vi "CreatePopupWindow.vi"(5 "Offset_y":i32, 6 "Flags (SDL_WINDOW_TOOLTIP)":T1=262144 items=["0"=0, "SDL_WINDOW_FULLSCREEN"=1, "SDL_WINDOW_OPENGL"=2, "SDL_WINDOW_OCCLUDED"=4, "SDL_WINDOW_HIDDEN"=8, "SDL_WINDOW_BORDERLESS"=16, "SDL_WINDOW_RESIZABLE"=32, "SDL_WINDOW_MINIMIZED"=64, "SDL_WINDOW_MAXIMIZED"=128, "SDL_WINDOW_MOUSE_GRABBED"=256, "SDL_WINDOW_INPUT_FOCUS"=512, "SDL_WINDOW_MOUSE_FOCUS"=1024, "SDL_WINDOW_EXTERNAL"=2048, "SDL_WINDOW_MODAL"=4096, "SDL_WINDOW_HIGH_PIXEL_DENSITY"=8192, "SDL_WINDOW_MOUSE_CAPTURE"=16384, "SDL_WINDOW_MOUSE_RELATIVE_MODE"=32768, "SDL_WINDOW_ALWAYS_ON_TOP"=65536, "SDL_WINDOW_UTILITY"=131072, "SDL_WINDOW_TOOLTIP"=262144, "SDL_WINDOW_POPUP_MENU"=524288, "SDL_WINDOW_KEYBOARD_GRABBED"=1048576, "SDL_WINDOW_VULKAN"=268435456, "SDL_WINDOW_METAL"=536870912, "SDL_WINDOW_TRANSPARENT"=1073741824, "SDL_WINDOW_NOT_FOCUSABLE"=2147483648], 7 "Offset_x":i32, 8 "No Error":errorcluster, 9 "H":i32, 10 "W":i32, 11 "Window [SDL_Window *]":i64) -> (0 "error out":errorcluster, 3 "Popup Window [SDL_Window *]":i64)   [LabVIEW 2024, in "SDL3.lvlib" / "Video.lvlib"]
doc: "<B>Summary</B>\nCreate a child popup window of the specified parent window.\n\n<B>Remarks</B>\nThe flags parameter must contain at least one of the following:\n\nSDL_WINDOW_TOOLTIP: The popup window is a tooltip and will not pass any input events.\nSDL_WINDOW_POPUP_MENU: The popup window is a popup menu. The topmost popup menu will implicitly gain the keyboard focus.\nThe following flags are not relevant to popup window creation and will be ignored:\n\nSDL_WINDOW_MINIMIZED\nSDL_WINDOW_MAXIMIZED\nSDL_WINDOW_FULLSCREEN\nSDL_WINDOW_BORDERLESS\nThe following flags are incompatible with popup window creation and will cause it to fail:\n\nSDL_WINDOW_UTILITY\nSDL_WINDOW_MODAL\nThe parent parameter must be non-null and a valid window. The parent of a popup window can be either a regular, toplevel window, or another popup window.\n\nPopup windows cannot be minimized, maximized, made fullscreen, raised, flash, be made a modal window, be the parent of a toplevel window, or grab the mouse and/or keyboard. Attempts to do so will fail.\n\nPopup windows implicitly do not have a border/decorations and do not appear on the taskbar/dock or in lists of windows such as alt-tab menus.\n\nIf a parent window is hidden or destroyed, any child popup windows will be recursively hidden or destroyed as well. Child popup windows not explicitly hidden will be restored when the parent is shown."
uses:
  Video.lvlib
  WindowFlags--ring.ctl
  Lib/SDL3-32.dll
  Error/Error.lvlib
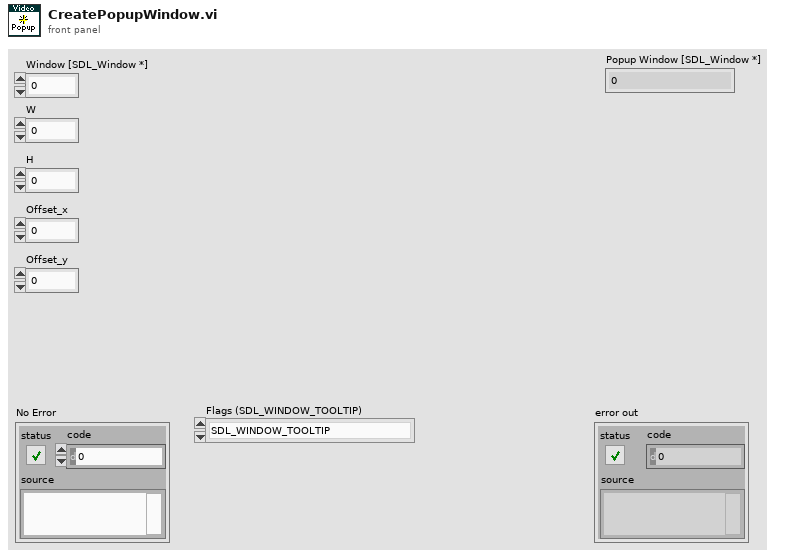
[diagram p1: front panel]
types:
  T1 = typedef "SDL3.lvlib/Video.lvlib/WindowFlags--ring.ctl" = u64
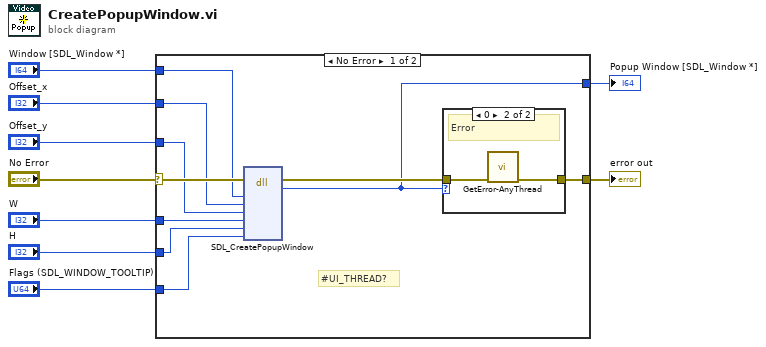
[diagram p0: block diagram]
diagram:
  n1 = case shown="No Error" "No Error" {
    selector: "No Error" -> [w18 w23]
    tunnel: "Flags (SDL_WINDOW_TOOLTIP)" -> [w19 _]
    tunnel: [w16 w23] -> w8
    tunnel: "W" -> [w15 _]
    tunnel: "H" -> [w14 _]
    tunnel: [w13 _] -> w5
    tunnel: "Window [SDL_Window *]" -> [w12 _]
    tunnel: "Offset_x" -> [w11 _]
    tunnel: "Offset_y" -> [w10 _]
    frame No Error {
      # "#UI_THREAD?"
      n2 = dll-call lib="C:/Users/Thomas/Documents/Projects/LV-SDL3/Lib/SDL3-*.*" fn="SDL_CreatePopupWindow"(error in=w18, "parent"=w12, "offset_x"=w11, "offset_y"=w10, "w"=w15, "h"=w14, "flags"=w19) -> (error out=w17:errorcluster, "return type"=w13:i64)  [unwired: 8 in, 1 out]
      n3 = case shown="0" w13 {
        tunnel: w17 -> [w20 w22]
        tunnel: [w20 w21] -> w16
        frame Default {
          # "Ok"
        }
        frame 0 {
          # "Error"
          n4 = call "GetError-AnyThread.vi"("No Error"=w22) -> ("error out"=w21:errorcluster)  [unwired: 10 in]
        }
      }
    }
    frame Error {
    }
  }
  "error out" <- w8
  "Popup Window [SDL_Window *]" <- w5
